vi "Microscope ID global.vi"() -> ()   [LabVIEW 2016]
panel:
  in  "Microscope ID":string="new-h-nu"
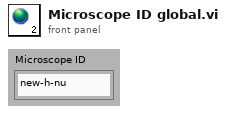
[diagram p1: front panel]
diagram:
